vi "Set Trigger Source.vi"(8 "error in (no error)":errorcluster, 10 "Trigger Source (Internal)":i32(ring) items=["Internal", "External rising edge", "External falling edge", "Single shot external rising edges", "Single shot external falling edges", "Single shot", "Line"], 11 "VISA resource name":refnum<visa-resource-name>) -> (0 "error out":errorcluster, 3 "VISA resource name out":refnum<visa-resource-name>, 4 "Device Errors":cluster{"code":i32, "Text":string}[](array[cluster]))   [LabVIEW 2014, in "Stanford Research DG645 - Driver.lvlib"]
doc: "Trigger Command: TSRC i\nInstrument Error Check\n\nSet the trigger source to i. The parameter i determines the trigger source according to the following table:\n\ni Trigger source\n0 Internal\n1 External rising edge\n2 External falling edge\n3 Single shot external rising edges\n4 Single shot external falling edges\n5 Single shot\n6 Line"
uses:
  Stanford Research DG645 - Driver.lvlib
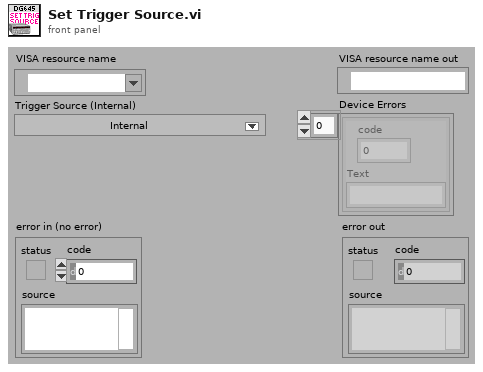
[diagram p1: front panel]
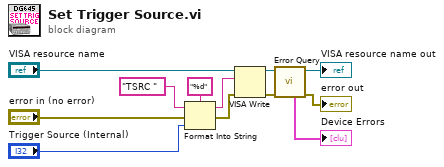
[diagram p0: block diagram]
diagram:
  n1 = Format Into String(format string="%d", initial string="TSRC " ("command"), error in="error in (no error)", "Trigger Source (Internal)") -> (resulting string=w3:string, error out=w2:errorcluster)
  n2 = VISA Write(VISA resource name="VISA resource name", write buffer=w3, error in (no error)=w2) -> (VISA resource name out=w9:refnum<visa-resource-name>, error out=w6:errorcluster)  [unwired: 1 out]
  n3 = call "Error Query.vi"("error in (no error)"=w6, "VISA resource name"=w9) -> ("error out"=→"error out":errorcluster, "VISA resource name out"=→"VISA resource name out":refnum<visa-resource-name>, "Device Errors"=→"Device Errors":cluster{"code":i32, "Text":string}[])  [unwired: 7 in]
